vi "From 2D Bool Tree Data.vi"(11 "Tree Data":refnum<class "Tree Data.lvclass">) -> (2 "2D Bool":bool[][](array[boolean]))   [LabVIEW 2017, in "Tree API.lvlib" / "2D Bool.lvclass"]
doc: "Extract a 2D Bool value from Tree Data type."
uses:
  2D Bool.lvclass
  Tree Data/Tree Data.lvclass
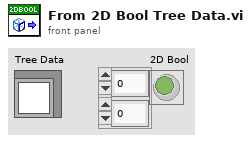
[diagram p1: front panel]
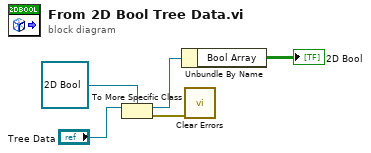
[diagram p0: block diagram]
diagram:
  n1 = To More Specific Class(target class=refnum<class "2D Bool.lvclass"> refnum ("Tree API.lvlib:2D Bool.lvclass"), reference="Tree Data") -> (specific class reference=w3:refnum<class "2D Bool.lvclass">, error out=w2:errorcluster)  [unwired: 1 in]
  n2 = Unbundle By Name(w3) -> ("Bool Array"=→"2D Bool":bool[][])
  n3 = call <vilib>:"Clear Errors.vi"("error in (no error)"=w2) -> ()  [unwired: 5 in, 2 out]
